vi "Read Mods.vi"(8 "error in (no error)":errorcluster, 11 "ControlKeyDownMsg in":refnum<class "ControlKeyDownMsg.lvclass">) -> (0 "error out":errorcluster, 2 "Mods":cluster{"Double Click":bool, "Menu Key":bool}, 3 "ControlKeyDownMsg out":refnum<class "ControlKeyDownMsg.lvclass">)   [LabVIEW 2018, in "MVA Framework.lvlib" / "ActorEvents.lvlib" / "ControlKeyDownMsg.lvclass"]
uses:
  ControlKeyDownMsg.lvclass
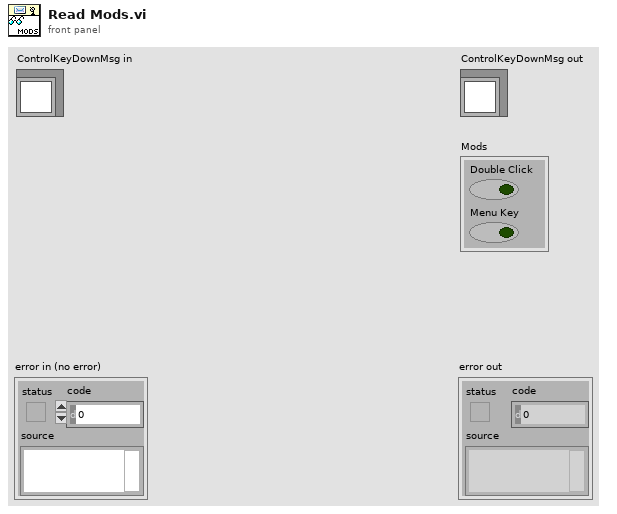
[diagram p1: front panel]
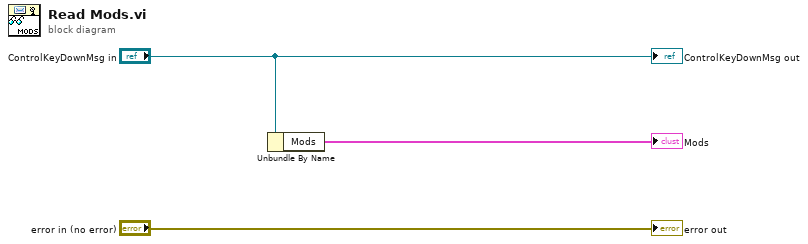
[diagram p0: block diagram]
diagram:
  n1 = Unbundle By Name("ControlKeyDownMsg in") -> ("Mods"=→"Mods":cluster{"Double Click":bool, "Menu Key":bool})
  "error out" <- "error in (no error)"
  "ControlKeyDownMsg out" <- "ControlKeyDownMsg in"
